vi "Send Text Message.vi"() -> ()   [LabVIEW 2015]
doc: "Demonstrates how to send an SMS text message to a phone number with the SNS VIs."
uses:
  Core/HTTP Request/Region.ctl
  Core/HTTP Request/AWS Credentials.ctl
  Phone Number/Phone Number.lvclass
  Core/HTTP Request/HTTP Request.lvclass
panel:
  in  "Message":string
  in  "Region":T1
  in  "Secret Key":string
  in  "Access Key":string
  in  "Phone Number":string
  # "Overview: Demonstrates how to send an SMS text message to a phone number with the SNS VIs.\nRequirements: LabVIEW AWS Toolkit and a registered Amazon AWS account\nInstructions:\n1. Specify the Access Key and Secret Key for your AWS account. You can create an account at http://aws.amazon.com.\n2. Specify a Phone Number for sending an SMS message. Note that the number must be in +1xxxyyyzzzz format.\n3. Run the VI. You should receive the specified message at the specified phone number within a few minutes."
  # "Note: The phone number must be in +1xxxyyyzzzz format, e.g. +15120123456"
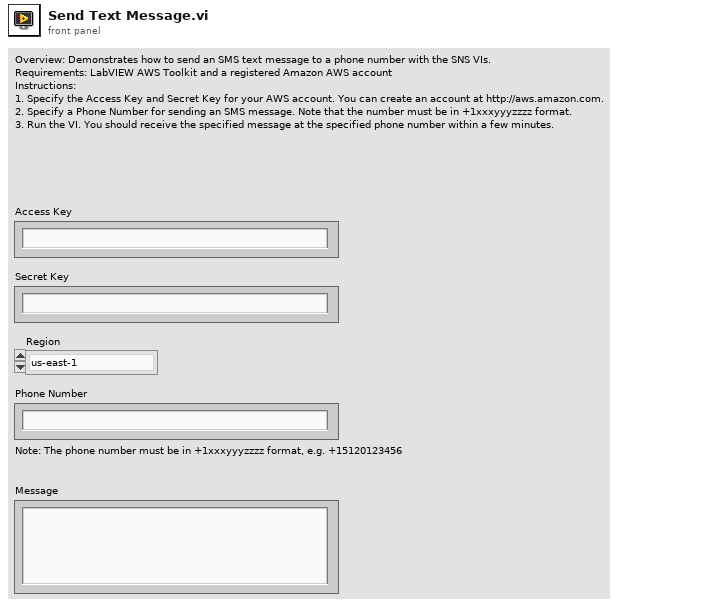
[diagram p1: front panel]
types:
  T1 = typedef "NI_AWS_Core.lvlib/HTTP Request.lvclass/Region.ctl" = enum16{"us-east-1", "us-east-2", "us-west-1", "us-west-2", "ap-northeast-1", "ap-northeast-2", "ap-southeast-1", "ap-southeast-2", "ca-central-1", "eu-central-1", "eu-west-1", "eu-west-2", "sa-east-1"}
  T2 = typedef "NI_AWS_Core.lvlib/HTTP Request.lvclass/AWS Credentials.ctl" = cluster{"Access Key":string, "Secret Key":string}
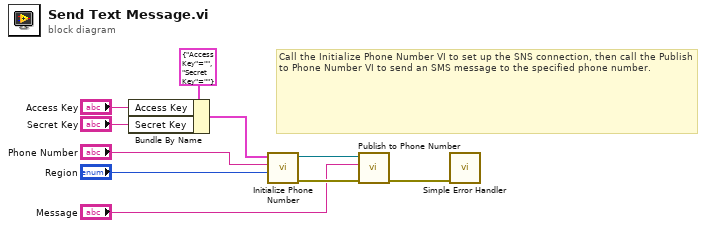
[diagram p0: block diagram]
diagram:
  # "Call the Initialize Phone Number VI to set up the SNS connection, then call the Publish to Phone Number VI to send an SMS message to the specified phone number."
  n1 = Bundle By Name(cluster=T2 {"Access Key"="", "Secret Key"=""} ("AWS Credentials"), "Access Key"="Access Key", "Secret Key"="Secret Key") -> (w4:T2)
  n2 = call "Initialize Phone Number.vi"("Region"="Region", "Phone Number"="Phone Number", "AWS Credentials"=w4) -> ("error out"=w9:errorcluster, "Phone Number"=w10:refnum<class "Phone Number.lvclass">)  [unwired: 7 in]
  n3 = call "Publish to Phone Number.vi"("error in (no error)"=w9, "Message"="Message", "Phone Number in"=w10) -> ("error out"=w8:errorcluster)  [unwired: 7 in, 1 out]
  n4 = call <vilib>:"Simple Error Handler.vi"("error in (no error)"=w8) -> ()  [unwired: 4 in, 5 out]
